vi "List Policies.vi"(8 "error in (no error)":errorcluster, 10 "Only Attached":bool, 11 "IAM Session in":refnum<class "IAM Session.lvclass">) -> (0 "error out":errorcluster, 2 "Policies":T1[](array[typedef]), 3 "IAM Session out":refnum<class "IAM Session.lvclass">)   [LabVIEW 2015, in "NI_AWS_IAM.lvlib" / "IAM Session.lvclass"]
uses:
  IAM Session.lvclass
  Policy.ctl
  Core/HTTP Request/Request Options.ctl
  Core/HTTP Request/Name Value Pair.ctl
  Core/HTTP Request/Region handling.ctl
  Core/HTTP Request/URL formatting.ctl
  Core/HTTP Request/HTTP Request.lvclass
  XML Parsing/NI_XML Parsing.lvlib
  NI_AWS_IAM.lvlib
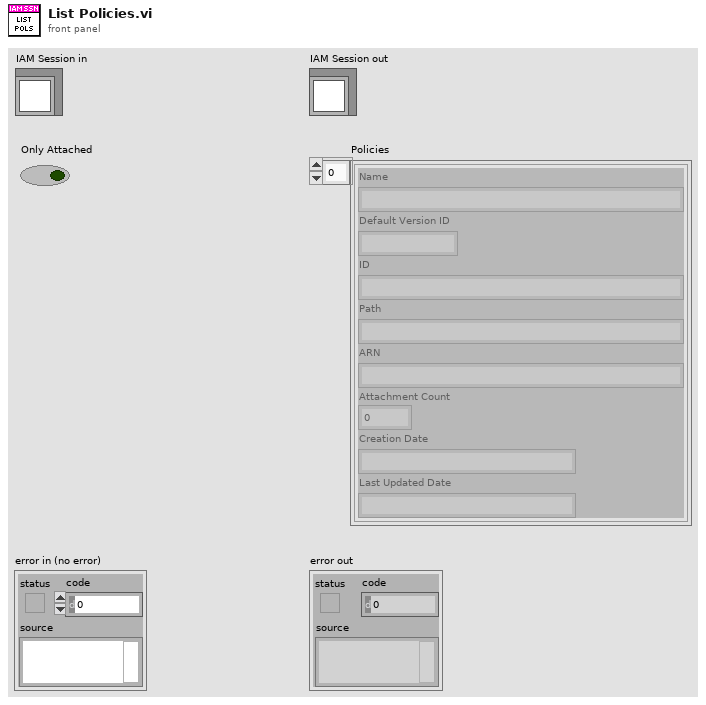
[diagram p1: front panel]
types:
  T1 = typedef "NI_AWS_IAM.lvlib/Policy.ctl" = cluster{"Name":string, "Default Version ID":string, "ID":string, "Path":string, "ARN":string, "Attachment Count":i32, "Creation Date":string, "Last Updated Date":string}
  T2 = typedef "NI_AWS_Core.lvlib/HTTP Request.lvclass/Name Value Pair.ctl" = cluster{"name":string, "value":string}
  T3 = typedef "NI_AWS_Core.lvlib/HTTP Request.lvclass/Request Options.ctl" = cluster{"request headers":T2[], "request parameters":T2[], "request body":string, "region handling":T4, "URL formatting":T5}
  T4 = typedef "NI_AWS_Core.lvlib/HTTP Request.lvclass/Region handling.ctl" = enum16{"use region everywhere", "use region (authentication only)", "use region (URL only)", "ignore region everwhere"}
  T5 = typedef "NI_AWS_Core.lvlib/HTTP Request.lvclass/URL formatting.ctl" = enum16{"region-", "region."}
  T6 = typedef "NI_AWS_Core.lvlib/HTTP Request.lvclass/Response.ctl" = cluster{"Headers":string, "Body":string}
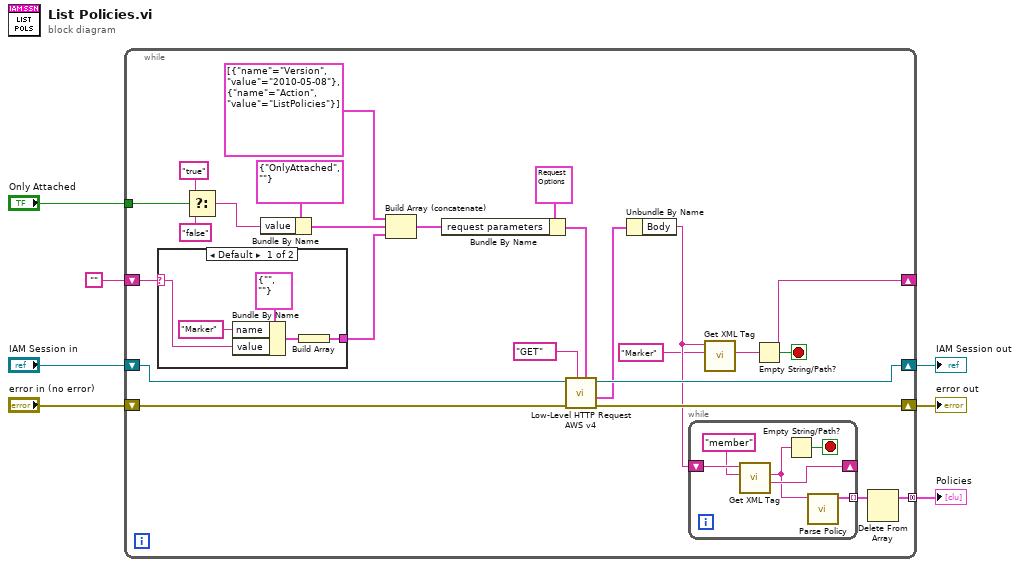
[diagram p0: block diagram]
diagram:
  n1 = while {
    shift-right: [w30] -> w6
    shift-left: "error in (no error)" -> [w31]
    shift-right: [w29] -> w5
    shift-left: "IAM Session in" -> [w28]
    shift-right: [w18] -> _
    shift-left: "" -> [w22]
    tunnel: [w15] -> w2 mode=concatenating
    tunnel: "Only Attached" -> [w11]
    stop <- w17 stop-if-true
    n2 = case shown="Default" w22 {
      selector: w22 -> [w34 _]
      tunnel: [w32 _] -> w21
      frame Default {
        n3 = Bundle By Name(cluster=T2 {"name"="", "value"=""} ("Name Value Pair"), "name"="Marker", "value"=w34) -> (w33:T2)
        n4 = Build Array(w33) -> (w32:T2[])
      }
      frame "" {
      }
    }
    n5 = Select(t="true", s=w11, f="false") -> (s? t:f=w8:string)
    n6 = Bundle By Name(cluster=T2 {"name"="OnlyAttached", "value"=""} ("Name Value Pair"), "value"=w8) -> (w12:T2)
    n7 = Build Array (concatenate)(T2[] [{"name"="Version", "value"="2010-05-08"}, {"name"="Action", "value"="ListPolicies"}], w12, w21) -> (w25:T2[])
    n8 = Bundle By Name(cluster=T3 {"request headers"=[], "request parameters"=[], "request body"="", "region handling"=enum."use region everywhere", "URL formatting"=enum."region."} ("Request Options"), "request parameters"=w25) -> (w26:T3)
    n9 = call "Low-Level HTTP Request AWS v4.vi"("Request Options"=w26, "HTTP-Verb"="GET", "error in (no error)"=w31, "AWS Core in"=w28) -> ("error out"=w30:errorcluster, "Response"=w23:T6, "AWS Core out"=w29:refnum<class "IAM Session.lvclass">)  [unwired: 4 in, 1 out]
    n10 = Unbundle By Name(w23) -> ("Body"=w20:string)
    n11 = while {
      shift-right: [w40] -> _
      shift-left: w20 -> [w42]
      tunnel: [w38] -> w16 mode=indexing
      stop <- w39 stop-if-true
      n12 = call "Get XML Tag.vi"("Tag name"="member", "XML String in"=w42) -> ("Remaining string"=w40:string, "Tag value"=w37:string)  [unwired: 5 in, 3 out]
      n13 = Empty String/Path?(string/path=w37) -> (empty?=w39:bool)
      n14 = call "Parse Policy.vi"("Response body"=w37) -> ("Policy"=w38:T1)  [unwired: 10 in]
    }
    n15 = call "Get XML Tag.vi"("Tag name"="Marker", "XML String in"=w20) -> ("Tag value"=w18:string)  [unwired: 5 in, 4 out]
    n16 = Empty String/Path?(string/path=w18) -> (empty?=w17:bool)
    n17 = Delete From Array(array=w16) -> (array with subset deleted=w15:T1[])  [unwired: 2 in, 1 out]
  }
  "error out" <- w6
  "IAM Session out" <- w5
  "Policies" <- w2
